vi "Step-3-Multiply-U64.vi"(10 "c[0]":u64=7208282044413215947 format="%.0x", 11 "b[0]":u64=11316410058078726994 format="%.0x") -> (2 "lo":u64=3283368253233308166 format="%.0x", 3 "hi":u64=7709959024924952286 format="%.0x")   [LabVIEW 2017]
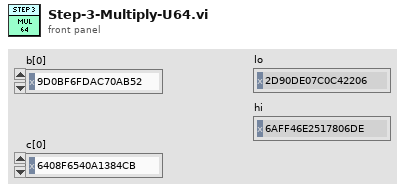
[diagram p1: front panel]
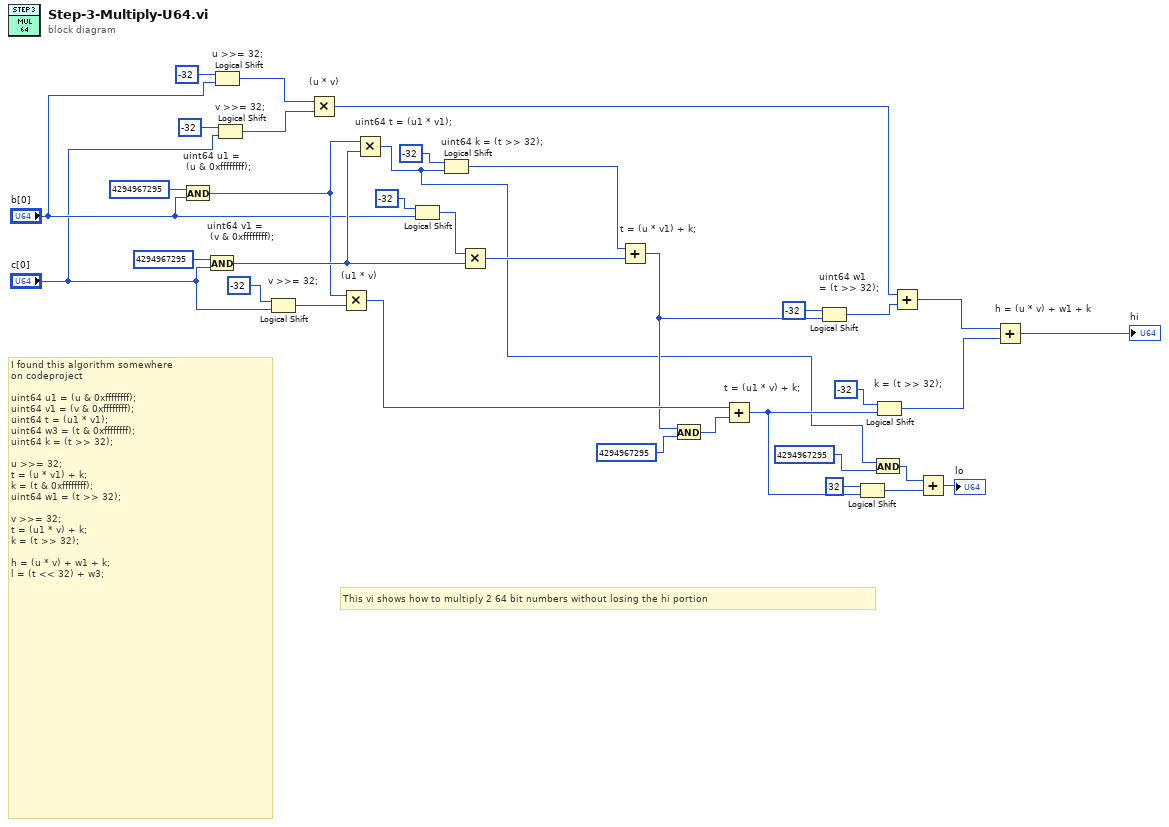
[diagram p0: block diagram]
diagram:
  # "This vi shows how to multiply 2 64 bit numbers without losing the hi portion"
  # "I found this algorithm somewhere\non codeproject\n\nuint64 u1 = (u & 0xffffffff);\nuint64 v1 = (v & 0xffffffff);\nuint64 t = (u1 * v1);\nuint64 w3 = (t & 0xffffffff);\nuint64 k = (t >> 32);\n\nu >>= 32;\nt = (u * v1) + k;\nk = (t & 0xffffffff);\nuint64 w1 = (t >> 32);\n\nv >>= 32;\nt = (u1 * v) + k;\nk = (t >> 32);\n\nh = (u * v) + w1 + k;\nl = (t << 32) + w3;"
  n1 = And "uint64 u1 =\n (u & 0xffffffff);"(x=u32 4294967295, y="b[0]") -> (x .and. y?=w27:u64)
  n2 = And "uint64 v1 =\n (v & 0xffffffff);"(x=u32 4294967295, y="c[0]") -> (x .and. y?=w32:u64)
  n3 = Logical Shift "u >>= 32;"(y=i16 -32, x="b[0]") -> (x << y=w15:u64)
  n4 = Logical Shift "v >>= 32;"(y=i16 -32, x="c[0]") -> (x << y=w14:u64)
  n5 = Logical Shift "v >>= 32;"(y=i16 -32, x="c[0]") -> (x << y=w24:u64)
  n6 = Multiply "(u * v)"(x=w15, y=w14) -> (x*y=w13:u64)
  n7 = Multiply "(u1 * v)"(x=w27, y=w24) -> (x*y=w22:u64)
  n8 = Multiply "uint64 t = (u1 * v1);"(x=w27, y=w32) -> (x*y=w5:u64)
  n9 = Logical Shift(y=i16 -32, x="b[0]") -> (x << y=w11:u64)
  n10 = Logical Shift "uint64 k = (t >> 32);"(y=i16 -32, x=w5) -> (x << y=w31:u64)
  n11 = Multiply(x=w11, y=w32) -> (x*y=w30:u64)
  n12 = Add "t = (u * v1) + k;"(x=w31, y=w30) -> (x+y=w19:u64)
  n13 = And(x=w19, y=u32 4294967295 ("x")) -> (x .and. y?=w21:u64)
  n14 = Add "t = (u1 * v) + k;"(x=w22, y=w21) -> (x+y=w10:u64)
  n15 = Logical Shift "uint64 w1 \n= (t >> 32);"(y=i16 -32, x=w19) -> (x << y=w18:u64)
  n16 = Logical Shift(y=i16 32, x=w10) -> (x << y=w8:u64)
  n17 = And(x=w5, y=u32 4294967295 ("x")) -> (x .and. y?=w7:u64)
  n18 = Logical Shift "k = (t >> 32);"(y=i16 -32, x=w10) -> (x << y=w26:u64)
  n19 = Add(x=w13, y=w18) -> (x+y=w28:u64)
  n20 = Add(x=w7, y=w8) -> (x+y=→"lo":u64)
  n21 = Add "h = (u * v) + w1 + k"(x=w28, y=w26) -> (x+y=→"hi":u64)
